vi "LSCI332 GetPID.vi"(6 "error in (no error)":errorcluster, 9 "Boucle(1)":u32(ring) caption="Boucle" items=["Boucle 1", "Boucle 2"], 10 "VISA Rsrc":refnum<visa-resource-name>="GPIB0::12::INSTR") -> (0 "error out":errorcluster, 3 "Paramètres PID":cluster{"P":dbl, "I":dbl, "D":i32}={"P"=1000.0, "I"=0.0, "D"=0} {"D" max=1000 step=1; "I" min=0.0 max=1000.0 step=0.1 format="%#.1f"; "P" min=0.0 max=1000.0 step=0.1 format="%#.1f"})   [LabVIEW 2019]
doc: "Ce VI envoie la commande Zone? au contrôlleur, ce qui retourne les paramètres de la zone spécifiée."
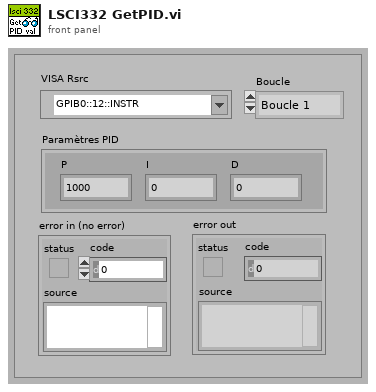
[diagram p1: front panel]
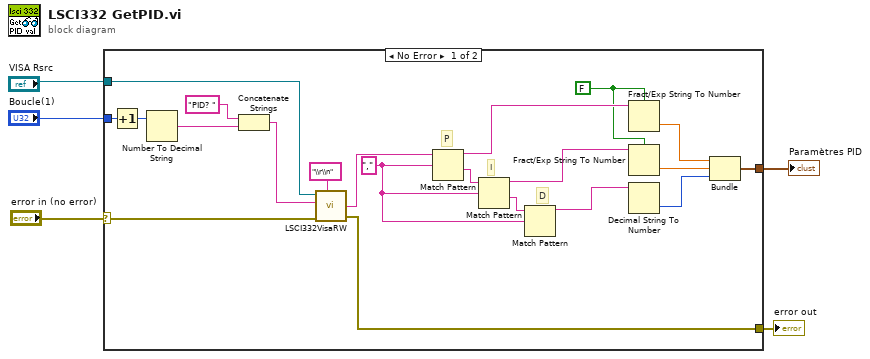
[diagram p0: block diagram]
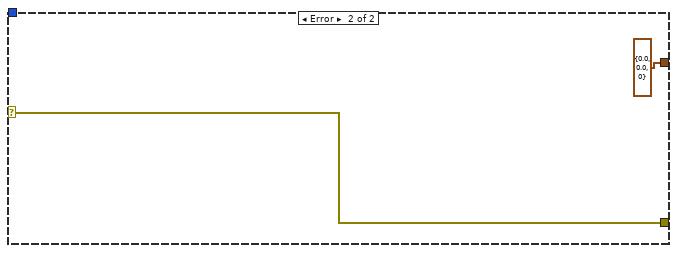
[diagram p2: hidden frame]
diagram:
  n1 = case shown="No Error" "error in (no error)" {
    selector: "error in (no error)" -> [w24 w28]
    tunnel: "VISA Rsrc" -> [w25 _]
    tunnel: "Boucle(1)" -> [w22 _]
    tunnel: [w23 w28] -> w3
    tunnel: [w7 cluster{dbl, dbl, i32} {0.0, 0.0, 0}] -> w1
    frame No Error {
      w6 = FALSE ("use system decimal point (T)")
      w17 = "," ("regular expression")
      # "D"
      # "I"
      # "P"
      n2 = Increment(x=w22) -> (x+1=w21:u32)
      n3 = Number To Decimal String(number=w21) -> (decimal integer string=w19:string)  [unwired: 1 in]
      n4 = Concatenate Strings("PID? " ("string"), w19) -> (w18:string)
      n5 = call <userlib>:"LSCI332VisaRW.vi"("error in (no error)"=w24, "EOS (Aucun)"="\\r\\n", "ChaineCom"=w18, "VISA Rsrc"=w25) -> ("error out"=w23:errorcluster, "ChaineRep"=w8:string)  [unwired: 3 in, 2 out]
      n6 = Match Pattern(string=w8, regular expression=w17) -> (before substring=w14:string, after substring=w16:string)  [unwired: 1 in, 2 out]
      n7 = Match Pattern(string=w16, regular expression=w17) -> (before substring=w13:string, after substring=w15:string)  [unwired: 1 in, 2 out]
      n8 = Match Pattern(string=w15, regular expression=w17) -> (before substring=w12:string)  [unwired: 1 in, 3 out]
      n9 = Fract/Exp String To Number(use system decimal point (T)=w6, string=w14) -> (number=w11:dbl)  [unwired: 2 in, 1 out]
      n10 = Fract/Exp String To Number(use system decimal point (T)=w6, string=w13) -> (number=w10:dbl)  [unwired: 2 in, 1 out]
      n11 = Decimal String To Number(string=w12) -> (number=w9:i32)  [unwired: 2 in, 1 out]
      n12 = Bundle(w11, w10, w9) -> (w7:cluster{dbl, dbl, i32})  [unwired: 1 in]
    }
    frame Error {
    }
  }
  "error out" <- w3
  "Paramètres PID" <- w1
